vi "Multicolumn_Listbox_Right-click select.vi"(6 "Disable when multiple selection":bool, 7 "Registered cell's string (hidden)":refnum<vi>, 8 "error in (no error)":errorcluster, 9 "Coords":T1, 10 "Button":u16, 11 "MulticolumnListbox in":refnum<vi>) -> (0 "error out":errorcluster, 3 "MulticolumnListbox out":refnum<vi>)   [LabVIEW 2020]
uses:
  <vilib>/Utility/miscctls.llb/LVPoint32TypeDef.ctl
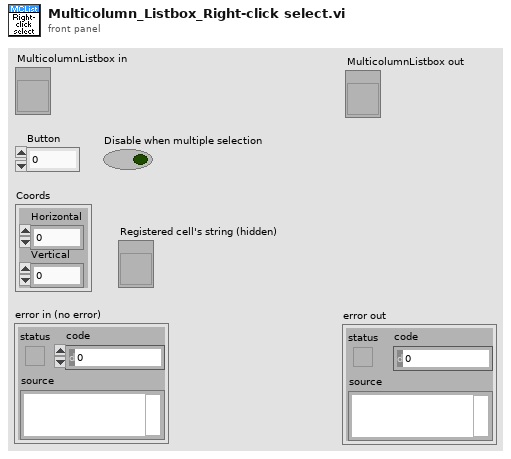
[diagram p1: front panel]
types:
  T1 = typedef "LVPoint32TypeDef.ctl" = cluster{"Horizontal":i32, "Vertical":i32}
  T2 = typedef "LVRowAndColumnTypeDef.ctl" = cluster{"Row":i32, "Column":i32}
  T3 = typedef "Test_Header_Info_MC_Listbox.ctl" = i32[]
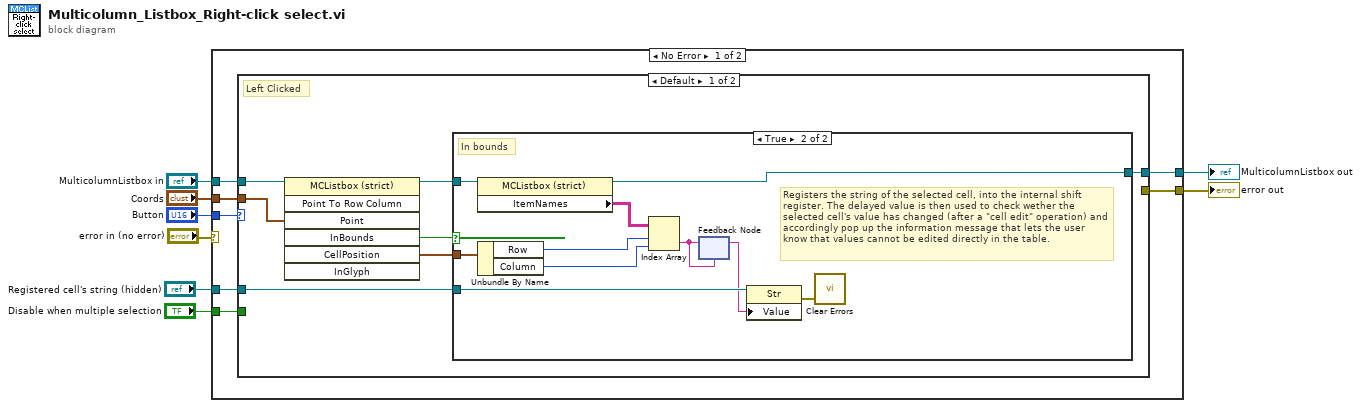
[diagram p0: block diagram]
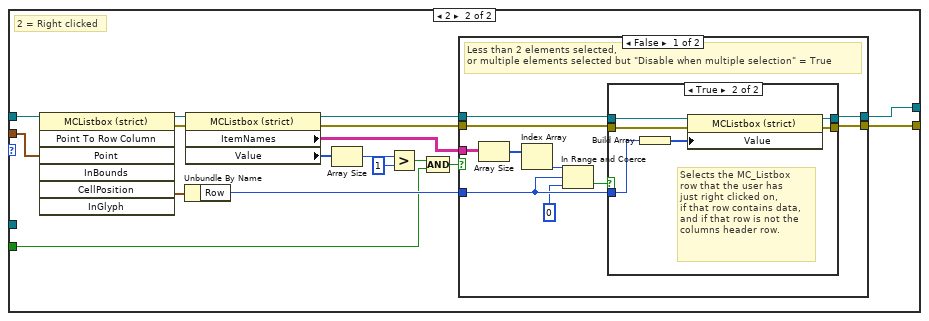
[diagram p3: hidden frame]
diagram:
  n1 = case shown="No Error" "error in (no error)" {
    selector: "error in (no error)" -> [_ w72]
    tunnel: "MulticolumnListbox in" -> [w15 w71]
    tunnel: "Coords" -> [w14 _]
    tunnel: "Button" -> [w13 _]
    tunnel: [w12 w72] -> w5
    tunnel: [w11 w71] -> w3
    tunnel: "Disable when multiple selection" -> [w10 _]
    tunnel: "Registered cell's string (hidden)" -> [w9 _]
    frame No Error {
      n2 = case shown="Default" w13 {
        tunnel: w14 -> [w21 w50]
        tunnel: w15 -> [w22 w49]
        tunnel: [_ w47] -> w12
        tunnel: [w18 w46] -> w11
        tunnel: w10 -> [_ w34]
        tunnel: w9 -> [w17 _]
        frame Default {
          # "Left Clicked"
          n3 = invoke on="Invoke Node" class="MCListbox (strict)" method="Point To Row Column"(reference=w22, "Point"=w21) -> (reference out=w19:refnum<vi>, "InBounds"=w16:bool, "CellPosition"=w20:T2)  [unwired: 5 in, 4 out]
          n4 = case shown="True" w16 {
            tunnel: w20 -> [_ w32]
            tunnel: w19 -> [w23 w29]
            tunnel: [w23 w28] -> w18
            tunnel: w17 -> [_ w27]
            frame False {
            }
            frame True {
              # "Registers the string of the selected cell, into the internal shift register. The delayed value is then used to check wether the selected cell's value has changed (after a \"cell edit\" operation) and accordingly pop up the information message that lets the user know that values cannot be edited directly in the table."
              # "In bounds"
              n5 = property class="MCListbox (strict)"(reference=w29) -> (reference out=w28:refnum<vi>, "ItemNames"=w33:string[][])  [unwired: 1 in, 1 out]
              n6 = Unbundle By Name(w32) -> ("Row"=w31:i32, "Column"=w30:i32)
              n7 = Index Array(array=w33, index (row)=w31, index (col)=w30) -> (element=w25:string)
              n8 = feedback-in #1(w25) -> ()
              n9 = feedback #1(w25) -> (w24:string)
              n10 = property on="Property Node" class="Str"(reference=w27, "Value"=w24) -> (error out=w26:errorcluster)  [unwired: 1 in, 1 out]
              n11 = call <vilib>:"Clear Errors.vi"("error in (no error)"=w26) -> ()  [unwired: 5 in, 2 out]
            }
          }
        }
        frame 2 {
          # "2 = Right clicked"
          n12 = invoke on="Invoke Node" class="MCListbox (strict)" method="Point To Row Column"(reference=w49, "Point"=w50) -> (reference out=w43:refnum<vi>, error out=w45:errorcluster, "CellPosition"=w48:T2)  [unwired: 5 in, 4 out]
          n13 = Unbundle By Name(w48) -> ("Row"=w40:i32)
          n14 = property class="MCListbox (strict)"(reference=w43, error in=w45) -> (reference out=w42:refnum<vi>, error out=w44:errorcluster, "ItemNames"=w41:string[][], "Value"=w39:T3)
          n15 = Array Size(array=w39) -> (size(s)=w38:i32)
          n16 = Greater?(x=w38, y=1) -> (0:w36:bool)
          n17 = Compound Arithmetic op=AND(w36, w34) -> (w35:bool)
          n18 = case shown="False" w35 {
            tunnel: [w60 w69] -> w47
            tunnel: [w59 w70] -> w46
            tunnel: w44 -> [w58 w69]
            tunnel: w42 -> [w57 w70]
            tunnel: w41 -> [w56 _]
            tunnel: w40 -> [w54 _]
            frame False {
              # "Less than 2 elements selected,\nor multiple elements selected but \"Disable when multiple selection\" = True"
              n19 = Array Size(array=w56) -> (size(s)=w55:i32[])
              n20 = Index Array(array=w55) -> (element=w52:i32)  [unwired: 1 in]
              n21 = In Range and Coerce(upper limit=w52, x=w54, lower limit=0) -> (In Range?=w51:bool)  [unwired: 1 out]
              n22 = case shown="True" w51 {
                tunnel: [w61 w67] -> w60
                tunnel: [w62 w66] -> w59
                tunnel: w58 -> [w61 w65]
                tunnel: w57 -> [w62 w64]
                tunnel: w54 -> [_ w63]
                frame False {
                }
                frame True {
                  # "Selects the MC_Listbox \nrow that the user has \njust right clicked on,\nif that row contains data,\nand if that row is not the columns header row."
                  n23 = Build Array(w63) -> (w68:i32[])
                  n24 = property class="MCListbox (strict)"(reference=w64, error in=w65, "Value"=w68) -> (reference out=w66:refnum<vi>, error out=w67:errorcluster)
                }
              }
            }
            frame True {
            }
          }
        }
      }
    }
    frame Error {
    }
  }
  "error out" <- w5
  "MulticolumnListbox out" <- w3
